vi "UHR-Fleezers Control (host) - 11.8.vi"() -> ()   [LabVIEW 2014] (continued)
        n1091 = Or(x="+ phase (APD Acq)", y="- phase (APD Acq)") -> (x .or. y?=w1470:bool)
        n1092 = xnode "Read/Write Control"("FPGA VI Reference In"=w1477, "error in"=w1476, "Phase Count Adjustment (APD Acq)"=w1474) -> ("FPGA VI Reference Out"=w1472:T19, "error out"=w1473:errorcluster)
        n1093 = xnode "Read/Write Control"("FPGA VI Reference In"=w1472, "error in"=w1473, "+ phase (APD Acq)"=w1470) -> ("error out"=w1471:errorcluster)  [unwired: 1 out]
      }
      event "Phase adj. (GI)", "+ phase (GI)", "- phase (GI)": Value Change {
        n1094 = event-data() -> ()  [unwired: 7 out]
        n1095 = Negate(x="Phase adj. (GI)") -> (-x=w1486:i16)
        n1096 = Select(t=w1486, s="+ phase (GI)", f="Phase adj. (GI)") -> (s? t:f=w1485:i16)
        n1097 = Or(x="+ phase (GI)", y="- phase (GI)") -> (x .or. y?=w1481:bool)
        n1098 = xnode "Read/Write Control"("FPGA VI Reference In"=w1488, "error in"=w1487, "Phase count adjustment (GI)"=w1485) -> ("FPGA VI Reference Out"=w1483:T19, "error out"=w1484:errorcluster)
        n1099 = xnode "Read/Write Control"("FPGA VI Reference In"=w1483, "error in"=w1484, "+ phase (GI)"=w1481) -> ("error out"=w1482:errorcluster)  [unwired: 1 out]
      }
      event "Phase adj. (GI) 2", "+ phase (GI) 2", "- phase (GI) 2": Value Change {
        n1100 = event-data() -> ()  [unwired: 7 out]
        n1101 = Negate(x="Phase adj. (GI) 2") -> (-x=w1497:i16)
        n1102 = Select(t=w1497, s="+ phase (GI) 2", f="Phase adj. (GI) 2") -> (s? t:f=w1496:i16)
        n1103 = Or(x="+ phase (GI) 2", y="- phase (GI) 2") -> (x .or. y?=w1492:bool)
        n1104 = xnode "Read/Write Control"("FPGA VI Reference In"=w1499, "error in"=w1498, "Phase count adjustment (GI) 2"=w1496) -> ("FPGA VI Reference Out"=w1494:T19, "error out"=w1495:errorcluster)
        n1105 = xnode "Read/Write Control"("FPGA VI Reference In"=w1494, "error in"=w1495, "+ phase (GI) 2"=w1492) -> ("error out"=w1493:errorcluster)  [unwired: 1 out]
      }
      event "Phase adj. (Green FB)", "- phase (Green FB)", "+ phase (Green FB)": Value Change {
        n1106 = event-data() -> ()  [unwired: 7 out]
        n1107 = Negate(x="Phase adj. (Green FB)") -> (-x=w1508:i16)
        n1108 = Select(t=w1508, s="+ phase (Green FB)", f="Phase adj. (Green FB)") -> (s? t:f=w1507:i16)
        n1109 = Or(x="+ phase (Green FB)", y="- phase (Green FB)") -> (x .or. y?=w1503:bool)
        n1110 = xnode "Read/Write Control"("FPGA VI Reference In"=w1510, "error in"=w1509, "Phase count adjustment (Green FB)"=w1507) -> ("FPGA VI Reference Out"=w1505:T19, "error out"=w1506:errorcluster)
        n1111 = xnode "Read/Write Control"("FPGA VI Reference In"=w1505, "error in"=w1506, "+ phase (Green FB)"=w1503) -> ("error out"=w1504:errorcluster)  [unwired: 1 out]
      }
      event "Invert APD Gate", "APD Gate ON Count", "APD Gate OFF Count", "APD Gate", "APD Integration Time (s)", "APD 1 AO Mult.", "APD 2 AO Mult.", "On one out of X cycles": Value Change {
        n1112 = event-data() -> ()  [unwired: 7 out]
        n1113 = Add(x="GI Frequency, ON count", y="GI Frequency, OFF count") -> (x+y=w1514:u32)
        n1114 = Add(x="APD Gate ON Count", y="APD Gate OFF Count") -> (x+y=w1527:u32)
        n1115 = Multiply(x="On one out of X cycles", y=w1514) -> (x*y=w1511:u32)
        "Green FB Count" <- w1511
        n1116 = Subtract(x=w1511, y="GI Frequency, ON count") -> (x-y=w1512:u32)
        n1117 = Multiply(x=w1527, y="On one out of X cycles") -> (x*y=w1526:u32)
        n1118 = Subtract(x=w1526, y="APD Gate ON Count") -> (x-y=w1525:u32)
        n1119 = local read "DMA Update Period (s)"() -> (w1528:dbl)
        n1120 = Multiply(x="APD Integration Time (s)", y=40000000.0) -> (x*y=w1533:dbl)
        n1121 = Reciprocal(x="APD Integration Time (s)") -> (1/x=→"APD Acq Rate (Hz)":dbl)
        n1122 = To Unsigned Long Integer(number=w1533) -> (unsigned 32bit integer=w1517:u32)
        "APD Int. Count" <- w1517
        n1123 = xnode "Read/Write Control"("FPGA VI Reference In"=w1537, "error in"=w1536, "Invert APD Gate"="Invert APD Gate", "APD Gate ON Count"="APD Gate ON Count", "APD Gate OFF Count"=w1525, "APD Acq Rate Count"=w1517, "APD Gate Operating Mode"="APD Gate", "APD 1 AO scale factor"="APD 1 AO Mult.", "APD 2 AO scale factor"="APD 2 AO Mult.", "Green interlace ON count"="GI Frequency, ON count", "Green interlace OFF count"=w1512, "Green interlace ON count 2"="GI Frequency, ON count", "Green interlace OFF count 2"=w1512, "Green FB Count"=w1511) -> ("error out"=w1535:errorcluster)  [unwired: 1 out]
        n1124 = Divide(x=w1528, y="APD Integration Time (s)") -> (x/y=w1531:dbl)
        n1125 = Multiply(x=2.0, y=w1531) -> (x*y=w1530:dbl)
        n1126 = local write "APD Samples/FIFO Acq."(w1531) -> ()
        n1127 = local write "APD Elements/DMA read"(w1530) -> ()
      }
      event "Number of F/B Scans (AOD)", "Scan Speed (nm/s)", "Scan BD", "Initial D (MHz)", "Step Size (nm)", "Scan Range (nm)", "Wiggle amp 1 (units?)": Value Change {
        w1599 = 123.0  # AOM cal (nm/MHz)
        n1128 = event-data() -> ()  [unwired: 7 out]
        n1129 = local read "BD 1 Frequency 1 (MHz)"() -> (w1582:dbl)
        n1130 = local read "AOM X Cal (nm/MHz)"() -> (w1574:dbl)
        n1131 = local read "BD 2 Frequency 1 (MHz)"() -> (w1588:dbl)
        n1132 = local read "X RF Frequency Limits (MHz)"() -> (w1586:T16)
        n1133 = local read "Y RF Frequency Limits (MHz)"() -> (w1583:T16)
        n1134 = Negate(x="Scan Range (nm)") -> (-x=w1552:dbl)
        n1135 = Divide(x=w1552, y=w1574) -> (x/y=w1556:dbl)
        n1136 = Select(t=w1586, s="Scan BD", f=w1583) -> (s? t:f=w1585:T16)
        n1137 = Select(t=w1582, s="Scan BD", f=w1588) -> (s? t:f=w1587:dbl)
        n1138 = Unbundle By Name(w1585) -> ("Maximum"=w1594:dbl, "Minimum"=w1593:dbl)
        n1139 = Add(x=w1556, y=w1587) -> (x+y=w1591:dbl)
        n1140 = Divide(x=w1552, y="Step Size (nm)") -> (x/y=w1571:dbl)
        n1141 = Divide(x="Step Size (nm)", y=w1574) -> (x/y=w1580:dbl)
        n1142 = Absolute Value(x=w1571) -> (abs(x)=w1555:dbl)
        n1143 = Sign(1:w1552) -> (0:w1553:dbl)
        n1144 = In Range and Coerce(upper limit=w1594, x=w1591, lower limit=w1593) -> (coerced(x)=w1590:dbl, In Range?=w1592:bool)
        n1145 = To Unsigned Quad Integer(1:w1555) -> (0:w1570:u64)
        "Scan steps (AOD)" <- w1570
        n1146 = call "IR AOM freq to word.vi"("Frequency In (MHz)"=w1580) -> ("Frequency Word Out (double)"=w1577:dbl)
        n1147 = Multiply(x=w1553, y=w1577) -> (x*y=w1554:dbl)
        n1148 = Subtract(x=w1591, y=w1590) -> (x-y=w1589:dbl)
        n1149 = To Quad Integer(1:w1554) -> (0:w1576:i64)
        "Incr. int (AOD)" <- w1576
        n1150 = Subtract(x=w1556, y=w1589) -> (x-y=w1575:dbl)
        "Scan Range (MHz)" <- w1575
        n1151 = Select(t=w1556, s=w1592, f=w1575) -> (s? t:f=w1595:dbl)
        n1152 = Multiply(x=w1575, y=w1574) -> (x*y=w1573:dbl)
        n1153 = Decrement(x=w1570) -> (x-1=w1623:u64)
        n1154 = Negate(x=w1573) -> (-x=w1569:dbl)
        n1155 = local write "Scan Range (nm)"(w1569) -> ()
        n1156 = Divide(x=w1595, y=w1623) -> (x/y=w1579:dbl)
        "Scan Increment (MHz)" <- w1579
        n1157 = call "IR AOM freq to word.vi"("Frequency In (MHz)"=w1579) -> ("Frequency Word Out (double)"=w1578:dbl)
        n1158 = Divide(x="Step Size (nm)", y="Scan Speed (nm/s)") -> (x/y=w1566:dbl)
        n1159 = To Quad Integer(1:w1578) -> ()  [unwired: 1 out]
        n1160 = local read "Number Interlace Sets"() -> (w1550:u8)
        n1161 = local read "AI Count (ticks)"() -> (w1551:u32)
        n1162 = local read "Total Counts (ticks)"() -> (w1549:u32)
        n1163 = local read "# Samples/trap"() -> (w1581:u32)
        n1164 = Multiply(x=w1551, y=w1550) -> (x*y=w1548:u32)
        n1165 = Divide(x=w1549, y=w1548) -> (x/y=w1547:dbl)
        n1166 = Select(t=w1582, s="Scan BD", f=w1588) -> (s? t:f=w1620:dbl)
        "Initial freq. (MHz)" <- w1620
        n1167 = Add(x=w1595, y=w1620) -> (x+y=→"Final freq. (MHz)":dbl)
        n1168 = Divide(x=w1549, y=40000000.0) -> (x/y=w1565:dbl)
        n1169 = Divide(x=w1566, y=w1565) -> (x/y=w1564:dbl)
        n1170 = To Unsigned Quad Integer(1:w1564) -> (0:w1539:u64)
        n1171 = Quotient & Remainder(x=w1539, y=u64 2) -> (x-y*floor(x/y)=w1543:u64)  [unwired: 1 out]
        n1172 = Equal?(x=w1543, y=u64 0) -> (x = y?=w1541:bool)
        n1173 = Decrement(x=w1539) -> (x-1=w1540:u64)
        n1174 = Select(t=w1539, s=w1541, f=w1540) -> (s? t:f=w1538:u64)
        "Cycles/step (AOD)" <- w1538
        n1175 = xnode "Read/Write Control"("FPGA VI Reference In"=w1631, "error in"=w1630, "Scan steps"=w1570, "Number of scans"="Number of F/B Scans (AOD)", "Cycles per step"=w1538, "Scan freq.  increment"=w1576, "Scan BD"="Scan BD") -> ("error out"=w1629:errorcluster)  [unwired: 1 out]
        n1176 = Multiply(x=w1570, y=w1538) -> (x*y=w1624:u64)
        n1177 = Multiply(x=w1624, y=u64 2) -> (x*y=w1546:u64)
        n1178 = Multiply(x=w1547, y=w1546) -> (x*y=w1545:dbl)
        "Data points/scan (f/b)" <- w1545
        n1179 = Multiply(x=w1545, y="Number of F/B Scans (AOD)") -> (x*y=w1627:dbl)
        "Data points/scans" <- w1627
        n1180 = Divide(x=w1627, y=w1581) -> (x/y=→"N sets should be saved":dbl)
        n1181 = Multiply(x=w1624, y=w1565) -> (x*y=w1563:dbl)
        "Time/Scan (s) (AOD)" <- w1563
        n1182 = Select(t=w1595, s="Scan BD", f=0.0) -> (s? t:f=w1621:dbl)
        n1183 = Select(t=0.0, s="Scan BD", f=w1595) -> (s? t:f=w1617:dbl)
        n1184 = local read "BD 2 Frequency 2 (MHz)"() -> (w1613:dbl)
        n1185 = local read "BD 1 Frequency 2 (MHz)"() -> (w1616:dbl)
        n1186 = Add(x=w1617, y=w1588) -> (x+y=w1614:dbl)
        n1187 = Add(x=w1582, y=w1621) -> (x+y=w1615:dbl)
        n1188 = Multiply(x=w1563, y=2.0) -> (x*y=w1562:dbl)
        n1189 = Multiply(x=w1562, y="Number of F/B Scans (AOD)") -> (x*y=w1559:dbl)
        n1190 = Divide(x=w1559, y=60.0) -> (x/y=→"Time to Finish All (min)":dbl)
        n1191 = Add(x="Trap 2 Bead Size (nm)", y="Trap 1 Bead Size (nm)") -> (x+y=w1603:dbl)
        n1192 = Divide(x=w1603, y=2.0) -> (x/y=w1597:dbl)
        n1193 = Subtract(x=w1614, y=w1613) -> (x-y=w1611:dbl)
        n1194 = Subtract(x=w1615, y=w1616) -> (x-y=w1612:dbl)
        n1195 = local read "Initial D (MHz)"() -> (w1600:dbl)
        n1196 = Square(x=w1611) -> (x^2=w1610:dbl)
        n1197 = Square(x=w1612) -> (x^2=w1609:dbl)
        n1198 = Add(x=w1609, y=w1610) -> (x+y=w1608:dbl)
        n1199 = Square Root(x=w1608) -> (sqrt(x)=w1607:dbl)
        "Final D (MHz)" <- w1607
        n1200 = Multiply(x=w1599, y=w1607) -> (x*y=w1606:dbl)
        n1201 = Multiply(x=w1600, y=w1599) -> (x*y=w1598:dbl)
        n1202 = Subtract(x=w1598, y=w1597) -> (x-y=→"Initial sep (nm)":dbl)
        n1203 = Subtract(x=w1606, y=w1597) -> (x-y=→"Final sep (nm)":dbl)
      }
      event "Freq or Amp switch first", "Swap F1 and F2", "Freq switch delay", "Amp switch delay": Value Change {
        n1204 = event-data() -> ()  [unwired: 7 out]
        n1205 = local read "Freq or Amp switch first"() -> (w1632:bool)
        n1206 = local read "Amp switch delay"() -> (w1633:u16)
        n1207 = local read "Freq switch delay"() -> (w1635:u16)
        n1208 = local read "Swap F1 and F2"() -> (w1634:bool)
        n1209 = xnode "Read/Write Control"("FPGA VI Reference In"=w1638, "error in"=w1637, "Freq switch delay"=w1635, "Swap F1 and F2"=w1634, "Amp switch delay"=w1633, "Freq or Amp switch first"=w1632) -> ("error out"=w1636:errorcluster)  [unwired: 1 out]
      }
      event "Scan steps (MCL)", "Number of scans (MCL)", "Scan Range (V)\n(of steps)", "2D or 1D Scan", "N APD Samp/step", "Fast Scan Dir", "Continuous MCL Scanning", "Scan lines (y)": Value Change {
        w1640 = 32767.0 ("y")
        n1210 = event-data() -> ()  [unwired: 7 out]
        n1211 = Select(t="Scan lines (y)", s="2D or 1D Scan", f="Number of scans (MCL)") -> (s? t:f=w1645:u64)
        n1212 = Decrement(x="Scan steps (MCL)") -> (x-1=w1661:u64)
        n1213 = Divide(x="Scan Range (V)\n(of steps)", y=w1661) -> (x/y=w1660:dbl)
        "Desired Scan Incr (V)" <- w1660
        n1214 = local read "APD Integration Time (s)"() -> (w1653:dbl)
        n1215 = Multiply(x=w1660, y=w1640) -> (x*y=w1669:dbl)
        n1216 = Divide(x=w1669, y=10.0) -> (x/y=w1659:dbl)
        "Desired incr (int)" <- w1659
        n1217 = local read "Update Count (MCL)"() -> (w1665:u32)
        n1218 = Round Toward -Infinity(1:w1659) -> (0:w1668:dbl)
        n1219 = To Word Integer(number=w1668) -> (16bit integer=w1643:i16)
        "Actual Incr. int (MCL)" <- w1643
        n1220 = Multiply(x=w1653, y=40000000.0) -> (x*y=w1666:dbl)
        n1221 = Divide(x=w1666, y=w1665) -> (x/y=w1664:dbl)
        n1222 = Multiply(x=i16 10, y=w1643) -> (x*y=w1641:i16)
        n1223 = Multiply(x="N APD Samp/step", y=w1664) -> (x*y=w1663:dbl)
        "Cycles/step (MCL)" <- w1663
        n1224 = Divide(x=w1641, y=w1640) -> (x/y=→"Actual MCL Inc (V)":dbl)
        n1225 = Multiply(x="N APD Samp/step", y="Scan steps (MCL)") -> (x*y=w1655:dbl)
        n1226 = local read "APD Samples/FIFO Acq."() -> (w1652:dbl)
        n1227 = Multiply(x=w1655, y=u64 2) -> (x*y=w1654:dbl)
        "Data points/scan (f+b)" <- w1654
        n1228 = Multiply(x=w1654, y=w1645) -> (x*y=w1672:dbl)
        "Data points/scans (MCL)" <- w1672
        n1229 = Multiply(x=w1653, y=w1654) -> (x*y=w1646:dbl)
        "Time/f+b scan (s) (MCL)" <- w1646
        n1230 = Divide(x=w1672, y=w1652) -> (x/y=→"N sets should be saved (MCL)":dbl)
        n1231 = Multiply(x=w1646, y=w1645) -> (x*y=→"Total Time (s)":dbl)
        n1232 = Not(x="Fast Scan Dir") -> (.not. x?=w1650:bool)
        n1233 = xnode "Read/Write Control"("FPGA VI Reference In"=w1676, "error in"=w1675, "Scan steps (MCL)"="Scan steps (MCL)", "Number of scans (MCL)"=w1645, "Cycles per step (MCL)"=w1663, "Scan freq.  increment (MCL)"=w1643, "1D or 2D Scan?"="2D or 1D Scan", "MCL Scan Axis"=w1650, "Cont. Scan (MCL)"="Continuous MCL Scanning") -> ("error out"=w1674:errorcluster)  [unwired: 1 out]
      }
      event "Read Cal": Value Change {
        w1678 = 1000.0 ("y")
        n1234 = event-data() -> ()  [unwired: 7 out]
        n1235 = local read "Save file name"() -> (w1703:path)
        n1236 = local write "Read Cal"(FALSE ("Read Cal")) -> ()
        n1237 = Strip Path(path=w1703) -> (stripped path=w1702:path)  [unwired: 1 out]
        n1238 = Path To String(path=w1702) -> (string=w1701:string)
        n1239 = Concatenate Strings(w1701, "\\current.cal" ("string")) -> (w1699:string)
        n1240 = String To Path(string=w1699) -> (path=w1698:path)
        n1241 = Open/Create/Replace File(file path (use dialog)=w1698, operation (0:open)=T25."open", access (0:read/write)=enum16{"read/write", "read-only", "write-only"}."read-only") -> (refnum out=w1706:refnum<file>, error out=w1692:errorcluster)  [unwired: 1 in, 3 out]
        n1242 = Deny Access(4:w1692, 7:w1706) -> (0:w1691:errorcluster, 3:w1697:refnum<file>)  [unwired: 1 out]
        n1243 = Read from Binary File(5:0.0, 8:w1691, 9:T24."big-endian, network order" ("byte order (0:big-endian, network order)"), 10:-1 ("count (1)"), 11:w1697) -> (0:w1690:errorcluster, 2:w1688:dbl[], 3:w1693:refnum<file>)  [unwired: 2 out]
        n1244 = Array To Cluster(array=w1688) -> (cluster=w1687:T27)
        n1245 = Unbundle(w1687) -> ("[0]"=w1686:dbl, "[1]"=w1685:dbl, "[2]"=w1684:dbl, "[3]"=w1683:dbl, "[4]"=w1682:dbl, "[5]"=w1681:dbl)
        n1246 = Close File(refnum=w1693, error in=w1690) -> (error out=→"Read cal error":errorcluster)  [unwired: 1 out]
        n1247 = Multiply(x=w1681, y=w1678) -> (x*y=w1679:dbl)
        n1248 = local write "T2 k_x (pN/nm)"(w1683) -> ()
        n1249 = local write "T1 k_x (pN/nm)"(w1684) -> ()
        n1250 = local write "T1 a_x (nm/V)"(w1686) -> ()
        n1251 = local write "T2 a_x (nm/V)"(w1685) -> ()
        n1252 = Multiply(x=w1682, y=w1678) -> (x*y=w1680:dbl)
        n1253 = local write "T1 offset_x (mV)"(w1680) -> ()
        n1254 = local write "T2 offset_x (mV)"(w1679) -> ()
      }
      event "Read FX file": Value Change {
        n1255 = event-data() -> ()  [unwired: 7 out]
        n1256 = local write "Read FX file"(FALSE ("Read residual")) -> ()
        n1257 = local read "Save file name"() -> (w1731:path)
        n1258 = Strip Path(path=w1731) -> (stripped path=w1730:path)  [unwired: 1 out]
        n1259 = Path To String(path=w1730) -> (string=w1729:string)
        n1260 = Concatenate Strings(w1729, "\\current.cal" ("string")) -> (w1727:string)
        n1261 = String To Path(string=w1727) -> (path=w1726:path)
        n1262 = Open/Create/Replace File(file path (use dialog)=w1726, operation (0:open)=T25."open", access (0:read/write)=enum16{"read/write", "read-only", "write-only"}."read-only") -> (refnum out=w1723:refnum<file>, error out=w1720:errorcluster)  [unwired: 3 in, 1 out]
        n1263 = Deny Access(4:w1720, 7:w1723) -> (0:w1719:errorcluster, 3:w1722:refnum<file>)  [unwired: 1 in]
        n1264 = Read from Binary File(5:0.0, 8:w1719, 9:T24."big-endian, network order" ("byte order (0:big-endian, network order)"), 10:-1 ("count"), 11:w1722) -> (0:w1715:errorcluster, 2:w1709:dbl[], 3:w1716:refnum<file>)  [unwired: 1 in, 1 out]
        n1265 = Index Array(array=w1709, index=6) -> (element=→"Bad fit error":dbl)
        n1266 = Index Array(array=w1709, index=7) -> (element=→"Fit offset":dbl)
        n1267 = Index Array(array=w1709, index=8) -> (element=→"Hyst. error":dbl)
        n1268 = Close File(refnum=w1716, error in=w1715) -> ()  [unwired: 2 out]
      }
      event "Abort MCL Scan": Value Change {
        n1269 = event-data() -> ()  [unwired: 7 out]
        n1270 = local write "MCL Scanning"(FALSE ("MCL Scanning")) -> ()
        n1271 = xnode "Read/Write Control"("FPGA VI Reference In"=w1736, "error in"=w1735, "Abort scan (MCL)"="Abort MCL Scan") -> ("error out"=w1734:errorcluster)  [unwired: 1 out]
      }
      event "Update Count (MCL)": Value Change {
        n1272 = event-data() -> ()  [unwired: 7 out]
        n1273 = xnode "Read/Write Control"("FPGA VI Reference In"=w1740, "error in"=w1739, "MCL count"="Update Count (MCL)") -> ("error out"=w1738:errorcluster)  [unwired: 1 out]
      }
      event "Phase adjust (MCL)", "+ phase (MCL)", "- phase (MCL)": Value Change {
        n1274 = event-data() -> ()  [unwired: 7 out]
        n1275 = Negate(x="Phase adjust (MCL)") -> (-x=w1749:i16)
        n1276 = Select(t=w1749, s="- phase (MCL)", f="Phase adjust (MCL)") -> (s? t:f=w1747:i16)
        n1277 = Or(x="- phase (MCL)", y="+ phase (MCL)") -> (x .or. y?=w1742:bool)
        n1278 = xnode "Read/Write Control"("FPGA VI Reference In"=w1751, "error in"=w1750, "Phase count adjustment (MCL)"=w1747) -> ("FPGA VI Reference Out"=w1743:T19, "error out"=w1744:errorcluster)
        n1279 = xnode "Read/Write Control"("FPGA VI Reference In"=w1743, "error in"=w1744, "+ phase (MCL)"=w1742) -> ("error out"=w1741:errorcluster)  [unwired: 1 out]
      }
      event "Abort AOD Scan": Value Change {
        n1280 = event-data() -> ()  [unwired: 7 out]
        n1281 = xnode "Read/Write Control"("FPGA VI Reference In"=w1755, "error in"=w1754, "Abort scan"="Abort AOD Scan") -> ("error out"=w1753:errorcluster)  [unwired: 1 out]
      }
      event "Continuous AOD Scanning": Value Change {
        n1282 = event-data() -> ()  [unwired: 7 out]
        n1283 = xnode "Read/Write Control"("FPGA VI Reference In"=w1759, "error in"=w1758, "Cont. Scan"="Continuous AOD Scanning") -> ("error out"=w1757:errorcluster)  [unwired: 1 out]
      }
      event "Index": Value Change {
        n1284 = event-data() -> ()  [unwired: 7 out]
        n1285 = call "Create new save file.vi"("Insert"="", "Ext"=".dat" ("string"), "Index In"="Index") -> ("Path Out"=→"Save file name":path, "Index Out"=w1760:dbl)
        "Save index" <- w1760
        n1286 = local write "Index"(w1760) -> ()
      }
      event "AO1", "AO2": Value Change {
        w1775 = 10.0 ("y")
        w1774 = 32767.0 ("y")
        n1287 = event-data() -> ()  [unwired: 7 out]
        n1288 = local read "AO2"() -> (w1773:dbl)
        n1289 = local read "AO1"() -> (w1770:dbl)
        n1290 = Multiply(x=w1770, y=w1774) -> (x*y=w1769:dbl)
        n1291 = Multiply(x=w1773, y=w1774) -> (x*y=w1772:dbl)
        n1292 = Divide(x=w1769, y=w1775) -> (x/y=w1768:dbl)
        n1293 = Divide(x=w1772, y=w1775) -> (x/y=w1771:dbl)
        n1294 = To Word Integer(number=w1768) -> (16bit integer=w1776:i16)
        n1295 = To Word Integer(number=w1771) -> (16bit integer=w1777:i16)
        n1296 = xnode "Read/Write Control"("FPGA VI Reference In"=w1767, "error in"=w1766, "AO1"=w1776, "AO2"=w1777) -> ("error out"=w1765:errorcluster)  [unwired: 1 out]
      }
      event "Inject Pump 1": Value Change {
        n1297 = event-data() -> ()  [unwired: 7 out]
        n1298 = local read "Use Harvard pumps\nfor beads (else Chemyx)"() -> (w1779:bool)
        n1299 = case shown="True" w1779 {
          tunnel: "Inject Pump 1" -> [w1783 w1821]
          tunnel: w1778 -> [_ w1822]
          frame False {
            n1300 = local read "Pump write delay (ms)"() -> (w1782:dbl)
            n1301 = local read "Chemyx Syringe Pump Serial Port"() -> (w1781:refnum<visa-resource-name>)
            n1302 = case shown="True" w1783 {
              tunnel: w1782 -> [w1789 w1803]
              tunnel: w1781 -> [w1786 w1802]
              frame False {
                n1303 = flat-sequence {
                  tunnel: w1786 -> [w1790]
                  tunnel: [w1790] -> w1787
                  tunnel: w1789 -> [_]
                  tunnel: [w1793] -> w1788
                  tunnel: w1787 -> [w1793]
                  tunnel: w1788 -> [w1794]
                  tunnel: [w1794] -> w1784
                  tunnel: [w1796] -> w1785
                  tunnel: w1784 -> [w1796]
                  tunnel: w1785 -> [w1798]
                  frame #0 {
                    n1304 = call "Write to pump.vi"("string"="enter pump1", "VISA resource name"=w1790) -> ()  [unwired: 1 out]
                  }
                  frame #1 {
                    n1305 = Wait (ms)(milliseconds to wait="Pump pause delay (ms)") -> ()  [unwired: 1 out]
                  }
                  frame #2 {
                    n1306 = call "Write to pump.vi"("string"="stop", "VISA resource name"=w1794) -> ()  [unwired: 1 out]
                  }
                  frame #3 {
                    n1307 = Wait (ms)(milliseconds to wait=u32 500) -> ()  [unwired: 1 out]
                  }
                  frame #4 {
                    n1308 = call "Write to pump.vi"("string"="stop", "VISA resource name"=w1798) -> ()  [unwired: 1 out]
                  }
                }
              }
              frame True {
                n1309 = flat-sequence {
                  tunnel: w1802 -> [w1812]
                  tunnel: w1803 -> [w1807]
                  tunnel: w1803 -> [w1814]
                  tunnel: w1802 -> [w1815]
                  tunnel: [w1815] -> w1800
                  tunnel: [w1817] -> w1801
                  tunnel: w1800 -> [w1817]
                  tunnel: w1801 -> [w1819]
                  frame #0 {
                    n1310 = local read "All Pump Parameters"() -> (w1806:T5)
                    n1311 = Unbundle By Name(w1806) -> ("Pump 1"=w1813:T28)
                    n1312 = call "Set pump parameters.vi"("Pump write delay (ms)"=w1807, "Volume (uL)"="Ch 1 Inject Volume (uL)", "Rate (uL/h)"="Ch 1 Inject Rate (ul/h)", "Units"=4.0, "Pump #"=1.0, "Pump Parameters In"=w1813, "VISA resource name"=w1812) -> ("Pump Parameters Out"=w1805:T28)  [unwired: 3 in]
                    n1313 = Bundle By Name(cluster=w1806, "Pump 1"=w1805) -> (w1804:T5)
                    n1314 = local write "All Pump Parameters"(w1804) -> ()
                  }
                  frame #1 {
                    n1315 = Wait (ms)(milliseconds to wait=w1814) -> ()  [unwired: 1 out]
                  }
                  frame #2 {
                    n1316 = call "Write to pump.vi"("string"="start", "VISA resource name"=w1815) -> ()  [unwired: 1 out]
                  }
                  frame #3 {
                    n1317 = Wait (ms)(milliseconds to wait=u32 500) -> ()  [unwired: 1 out]
                  }
                  frame #4 {
                    n1318 = call "Write to pump.vi"("string"="start", "VISA resource name"=w1819) -> ()  [unwired: 1 out]
                  }
                }
              }
            }
          }
          frame True {
            n1319 = case shown="True" w1821 {
              tunnel: w1822 -> [w1823 w1833]
              frame False {
                n1320 = flat-sequence {
                  tunnel: w1823 -> [w1825]
                  frame #0 {
                    n1321 = local write "Flushing P1"(FALSE ("Flushing P1")) -> ()
                    n1322 = Concatenate Strings("stop" ("string"), "\r") -> (w1827:string)
                    n1323 = VISA Write(VISA resource name=w1825, write buffer=w1827) -> ()  [unwired: 1 in, 3 out]
                  }
                  frame #1 {
                    n1324 = property on="Clear Volume P1" class="Bool (strict)"("Val(Sgnl)"=TRUE ("Value (Signaling)")) -> ()  [unwired: 2 in, 2 out]
                  }
                }
              }
              frame True {
                n1325 = local read "Normal Flow Rate (ul/h) P1"() -> (w1831:dbl)
                n1326 = Number To Decimal String(number=w1831) -> (decimal integer string=w1837:string)  [unwired: 1 in]
                n1327 = Concatenate Strings("irate  " ("string"), w1837, " u/h" ("string"), "\r") -> (w1835:string)
                n1328 = VISA Write(VISA resource name=w1833, write buffer=w1835) -> (VISA resource name out=w1832:refnum<visa-resource-name>)  [unwired: 1 in, 2 out]
                n1329 = Concatenate Strings("irun" ("string"), "\r") -> (w1839:string)
                n1330 = VISA Write(VISA resource name=w1832, write buffer=w1839) -> ()  [unwired: 1 in, 3 out]
              }
            }
          }
        }
      }
      event "Inject Pump 3": Value Change {
        n1331 = event-data() -> ()  [unwired: 7 out]
        n1332 = local read "Use Harvard pumps\nfor beads (else Chemyx)"() -> (w1842:bool)
        n1333 = case shown="True" w1842 {
          tunnel: "Inject Pump 3" -> [w1846 w1885]
          tunnel: w1841 -> [_ w1884]
          frame False {
            n1334 = local read "Pump write delay (ms)"() -> (w1845:dbl)
            n1335 = case shown="True" w1846 {
              tunnel: w1845 -> [w1852 w1866]
              tunnel: "Chemyx Syringe Pump Serial Port" -> [w1849 w1865]
              frame False {
                n1336 = flat-sequence {
                  tunnel: w1849 -> [w1853]
                  tunnel: [w1853] -> w1850
                  tunnel: w1852 -> [_]
                  tunnel: [w1856] -> w1851
                  tunnel: w1850 -> [w1856]
                  tunnel: w1851 -> [w1857]
                  tunnel: [w1857] -> w1847
                  tunnel: [w1859] -> w1848
                  tunnel: w1847 -> [w1859]
                  tunnel: w1848 -> [w1861]
                  frame #0 {
                    n1337 = call "Write to pump.vi"("string"="enter pump3", "VISA resource name"=w1853) -> ()  [unwired: 1 out]
                  }
                  frame #1 {
                    n1338 = local read "Pump pause delay (ms)"() -> (w1855:u32)
                    n1339 = Wait (ms)(milliseconds to wait=w1855) -> ()  [unwired: 1 out]
                  }
                  frame #2 {
                    n1340 = call "Write to pump.vi"("string"="stop", "VISA resource name"=w1857) -> ()  [unwired: 1 out]
                  }
                  frame #3 {
                    n1341 = Wait (ms)(milliseconds to wait=u32 0) -> ()  [unwired: 1 out]
                  }
                  frame #4 {
                    n1342 = call "Write to pump.vi"("string"="stop", "VISA resource name"=w1861) -> ()  [unwired: 1 out]
                  }
                }
              }
              frame True {
                n1343 = flat-sequence {
                  tunnel: w1865 -> [w1875]
                  tunnel: w1866 -> [w1870]
                  tunnel: w1866 -> [w1877]
                  tunnel: w1865 -> [w1878]
                  tunnel: [w1878] -> w1864
                  tunnel: [w1881] -> w1863
                  tunnel: w1864 -> [w1881]
                  tunnel: w1863 -> [w1882]
                  frame #0 {
                    n1344 = local read "All Pump Parameters"() -> (w1869:T5)
                    n1345 = Unbundle By Name(w1869) -> ("Pump 3"=w1876:T28)
                    n1346 = call "Set pump parameters.vi"("Pump write delay (ms)"=w1870, "Volume (uL)"="Ch 3 Inject Volume (uL)", "Rate (uL/h)"="Ch 3 Inject Rate (ul/h)", "Units"=4.0, "Pump #"=3.0, "Pump Parameters In"=w1876, "VISA resource name"=w1875) -> ("Pump Parameters Out"=w1868:T28)  [unwired: 3 in]
                    n1347 = Bundle By Name(cluster=w1869, "Pump 3"=w1868) -> (w1867:T5)
                    n1348 = local write "All Pump Parameters"(w1867) -> ()
                  }
                  frame #1 {
                    n1349 = Wait (ms)(milliseconds to wait=w1877) -> ()  [unwired: 1 out]
                  }
                  frame #2 {
                    n1350 = call "Write to pump.vi"("string"="start", "VISA resource name"=w1878) -> ()  [unwired: 1 out]
                  }
                  frame #3 {
                    n1351 = Wait (ms)(milliseconds to wait=u32 500) -> ()  [unwired: 1 out]
                  }
                  frame #4 {
                    n1352 = call "Write to pump.vi"("string"="start", "VISA resource name"=w1882) -> ()  [unwired: 1 out]
                  }
                }
              }
            }
          }
          frame True {
            n1353 = case shown="True" w1885 {
              tunnel: w1884 -> [w1886 w1893]
              frame False {
                n1354 = flat-sequence {
                  tunnel: w1886 -> [w1888]
                  frame #0 {
                    n1355 = local write "Flushing P3"(FALSE ("Flushing P3")) -> ()
                    n1356 = Concatenate Strings("stop" ("string"), "\r") -> (w1890:string)
                    n1357 = VISA Write(VISA resource name=w1888, write buffer=w1890) -> ()  [unwired: 1 in, 3 out]
                  }
                  frame #1 {
                    n1358 = property on="Clear Volume P3" class="Bool (strict)"("Val(Sgnl)"=TRUE ("Value (Signaling)")) -> ()  [unwired: 2 in, 2 out]
                  }
                }
              }
              frame True {
                n1359 = local read "Normal Flow Rate (ul/h) P3"() -> (w1894:dbl)
                n1360 = Number To Decimal String(number=w1894) -> (decimal integer string=w1900:string)  [unwired: 1 in]
                n1361 = Concatenate Strings("irate  " ("string"), w1900, " u/h" ("string"), "\r") -> (w1898:string)
                n1362 = VISA Write(VISA resource name=w1893, write buffer=w1898) -> (VISA resource name out=w1896:refnum<visa-resource-name>)  [unwired: 1 in, 2 out]
                n1363 = Concatenate Strings("irun" ("string"), "\r") -> (w1902:string)
                n1364 = VISA Write(VISA resource name=w1896, write buffer=w1902) -> ()  [unwired: 1 in, 3 out]
              }
            }
          }
        }
      }
      event "Inject Pump 2": Value Change {
        n1365 = event-data() -> ()  [unwired: 7 out]
        n1366 = local read "Pump write delay (ms)"() -> (w1906:dbl)
        n1367 = local read "Chemyx Syringe Pump Serial Port"() -> (w1904:refnum<visa-resource-name>)
        n1368 = flat-sequence {
          tunnel: w1904 -> [w1919]
          tunnel: w1906 -> [w1915]
          tunnel: "Inject Pump 2" -> [_]
          tunnel: w1906 -> [w1921]
          tunnel: w1904 -> [w1922]
          frame #0 {
            n1369 = local read "All Pump Parameters"() -> (w1914:T5)
            n1370 = Multiply(x=60.0, y="Flush Center Ch Rate (ul/m)") -> (x*y=w1911:dbl)
            n1371 = Unbundle By Name(w1914) -> ("Pump 2"=w1920:T28)
            n1372 = call "Set pump parameters.vi"("Pump write delay (ms)"=w1915, "Volume (uL)"="Flush Center Ch Volume (uL)", "Rate (uL/h)"=w1911, "Units"=3.0, "Pump #"=2.0, "Pump Parameters In"=w1920, "VISA resource name"=w1919) -> ("Pump Parameters Out"=w1913:T28)  [unwired: 3 in]
            n1373 = Bundle By Name(cluster=w1914, "Pump 2"=w1913) -> (w1912:T5)
            n1374 = Add(x="Flush Center Ch Volume (uL)", y="Total Volume\nFlushed (uL)") -> (x+y=w1908:dbl)
            n1375 = local write "All Pump Parameters"(w1912) -> ()
            n1376 = local write "Total Volume\nFlushed (uL)"(w1908) -> ()
          }
          frame #1 {
            n1377 = Wait (ms)(milliseconds to wait=w1921) -> ()  [unwired: 1 out]
          }
          frame #2 {
            n1378 = call "Write to pump.vi"("string"="start", "VISA resource name"=w1922) -> ()  [unwired: 1 out]
          }
        }
      }
      event "Sample Channel\nFlow": Value Change {
        n1379 = event-data() -> ()  [unwired: 7 out]
        n1380 = case shown="True" "Sample Channel\nFlow" {
          tunnel: w1925 -> [w1926 w1932]
          frame False {
            n1381 = flat-sequence {
              tunnel: w1926 -> [w1928]
              frame #0 {
                n1382 = local write "Flushing samp"(FALSE ("Flushing samp")) -> ()
                n1383 = Concatenate Strings("stop" ("string"), "\r") -> (w1931:string)
                n1384 = VISA Write(VISA resource name=w1928, write buffer=w1931) -> ()  [unwired: 1 in, 3 out]
              }
            }
          }
          frame True {
            n1385 = local read "Normal Flow rate (mL/h)"() -> (w1942:dbl)
            n1386 = Number To Decimal String(number=w1942) -> (decimal integer string=w1941:string)  [unwired: 1 in]
            n1387 = Concatenate Strings("irate " ("string"), w1941, " u/h" ("string"), "\r") -> (w1937:string)
            n1388 = VISA Write(VISA resource name=w1932, write buffer=w1937) -> (VISA resource name out=w1936:refnum<visa-resource-name>)  [unwired: 1 in, 2 out]
            n1389 = Concatenate Strings("irun" ("string"), "\r") -> (w1933:string)
            n1390 = VISA Write(VISA resource name=w1936, write buffer=w1933) -> ()  [unwired: 1 in, 3 out]
          }
        }
      }
      event "Start Flow": Value Change {
        n1391 = event-data() -> ()  [unwired: 7 out]
        n1392 = local write "Sample Channel\nFlow"(TRUE ("Sample Channel\nFlow")) -> ()
        n1393 = local write "Start Flow"(FALSE ("Start Flow")) -> ()
        n1394 = Concatenate Strings("irun" ("string"), "\r") -> (w1947:string)
        n1395 = VISA Write(VISA resource name=w1943, write buffer=w1947) -> ()  [unwired: 1 in, 3 out]
      }
      event "Stop Flow": Value Change {
        w1949 = FALSE ("Stop Flow")
        n1396 = event-data() -> ()  [unwired: 7 out]
        n1397 = local write "Stop Flow"(w1949) -> ()
        n1398 = local write "Sample Channel\nFlow"(w1949) -> ()
        n1399 = Concatenate Strings("stop" ("string"), "\r") -> (w1952:string)
        n1400 = VISA Write(VISA resource name=w1950, write buffer=w1952) -> ()  [unwired: 1 in, 3 out]
      }
      event "Normal Flow rate (mL/h)": Value Change {
        n1401 = event-data() -> ()  [unwired: 7 out]
        n1402 = Number To Decimal String(number="Normal Flow rate (mL/h)") -> (decimal integer string=w1959:string)  [unwired: 1 in]
        n1403 = Concatenate Strings("irate  " ("string"), w1959, " u/h" ("string"), "\r") -> (w1958:string)
        n1404 = VISA Write(VISA resource name=w1955, write buffer=w1958) -> ()  [unwired: 1 in, 3 out]
      }
      event "Flush Sample": Value Change {
        n1405 = event-data() -> ()  [unwired: 7 out]
        n1406 = flat-sequence {
          tunnel: w1961 -> [w1989]
          frame #0 {
            # "set parameters (rate, volume) for flush, clear volume"
            n1407 = Number To Decimal String(number="Flush rate (mL/m)") -> (decimal integer string=w1985:string)  [unwired: 1 in]
            n1408 = local write "Sample Channel\nFlow"(TRUE ("Sample Channel\nFlow")) -> ()
            n1409 = Concatenate Strings("irate  " ("string"), w1985, " u/m" ("string"), "\r") -> (w1987:string)
            n1410 = VISA Write(VISA resource name=w1989, write buffer=w1987) -> (VISA resource name out=w1983:refnum<visa-resource-name>)  [unwired: 1 in, 2 out]
            n1411 = Number To Decimal String(number="Flush volume (mL)") -> (decimal integer string=w1974:string)  [unwired: 1 in]
            n1412 = Reciprocal(x="Flush rate (mL/m)") -> (1/x=w1968:dbl)
            n1413 = Concatenate Strings("tvolume  " ("string"), w1974, " u" ("string"), "\r") -> (w1972:string)
            n1414 = Multiply(x=w1968, y="Flush volume (mL)") -> (x*y=w1966:dbl)
            n1415 = VISA Write(VISA resource name=w1983, write buffer=w1972) -> (VISA resource name out=w1971:refnum<visa-resource-name>)  [unwired: 1 in, 2 out]
            n1416 = Multiply(x=w1966, y=60.0) -> (x*y=→"Samp Flush Time (s)":dbl)
            n1417 = Concatenate Strings("cvolume" ("string"), "\r") -> (w1970:string)
            n1418 = VISA Write(VISA resource name=w1971, write buffer=w1970) -> (VISA resource name out=w1981:refnum<visa-resource-name>)  [unwired: 1 in, 2 out]
            n1419 = Concatenate Strings("irun" ("string"), "\r") -> (w1979:string)
            n1420 = VISA Write(VISA resource name=w1981, write buffer=w1979) -> ()  [unwired: 1 in, 3 out]
          }
          frame #1 {
            "Flushing samp" <- TRUE ("Boolean")
          }
        }
      }
      event "Flush Pump 3": Value Change {
        n1421 = event-data() -> ()  [unwired: 7 out]
        n1422 = flat-sequence {
          tunnel: w1991 -> [w1994]
          frame #0 {
            # "set paramaters (rate, volume) for flush, clear volume"
            n1423 = Number To Decimal String(number="Flush rate (uL/m) P3") -> (decimal integer string=w2016:string)  [unwired: 1 in]
            n1424 = local write "Inject Pump 3"(TRUE ("Inject Pump 3")) -> ()
            n1425 = Concatenate Strings("irate  " ("string"), w2016, " u/m" ("string"), "\r") -> (w2018:string)
            n1426 = VISA Write(VISA resource name=w1994, write buffer=w2018) -> (VISA resource name out=w2014:refnum<visa-resource-name>)  [unwired: 1 in, 2 out]
            n1427 = Reciprocal(x="Flush rate (uL/m) P3") -> (1/x=w1998:dbl)
            n1428 = Number To Decimal String(number="Volume (uL) P3") -> (decimal integer string=w2005:string)  [unwired: 1 in]
            n1429 = Multiply(x="Volume (uL) P3", y=w1998) -> (x*y=w1997:dbl)
            n1430 = Concatenate Strings("tvolume  " ("string"), w2005, " u" ("string"), "\r") -> (w2003:string)
            n1431 = Multiply(x=w1997, y=60.0) -> (x*y=→"HP3 Flush Time (s)":dbl)
            n1432 = VISA Write(VISA resource name=w2014, write buffer=w2003) -> (VISA resource name out=w2002:refnum<visa-resource-name>)  [unwired: 1 in, 2 out]
            n1433 = Concatenate Strings("cvolume" ("string"), "\r") -> (w2001:string)
            n1434 = VISA Write(VISA resource name=w2002, write buffer=w2001) -> (VISA resource name out=w2012:refnum<visa-resource-name>)  [unwired: 1 in, 2 out]
            n1435 = Concatenate Strings("irun" ("string"), "\r") -> (w2010:string)
            n1436 = VISA Write(VISA resource name=w2012, write buffer=w2010) -> ()  [unwired: 1 in, 3 out]
          }
          frame #1 {
            "Flushing P3" <- TRUE ("Flushing P3")
          }
        }
      }
      event "Flush Pump 1": Value Change {
        n1437 = event-data() -> ()  [unwired: 7 out]
        n1438 = flat-sequence {
          tunnel: [w2032] -> w2022
          tunnel: w2021 -> [w2025]
          tunnel: w2022 -> [_]
          frame #0 {
            # "set paramaters (rate, volume) for flush, clear volume"
            n1439 = local write "Inject Pump 1"(TRUE ("Inject Pump 1")) -> ()
            n1440 = Number To Decimal String(number="Flush rate (uL/m) P1") -> (decimal integer string=w2048:string)  [unwired: 1 in]
            n1441 = Concatenate Strings("irate  " ("string"), w2048, " u/m" ("string"), "\r") -> (w2050:string)
            n1442 = VISA Write(VISA resource name=w2025, write buffer=w2050) -> (VISA resource name out=w2046:refnum<visa-resource-name>)  [unwired: 1 in, 2 out]
            n1443 = Reciprocal(x="Flush rate (uL/m) P1") -> (1/x=w2029:dbl)
            n1444 = Number To Decimal String(number="Volume (uL) P1") -> (decimal integer string=w2037:string)  [unwired: 1 in]
            n1445 = Multiply(x="Volume (uL) P1", y=w2029) -> (x*y=w2028:dbl)
            n1446 = Concatenate Strings("tvolume  " ("string"), w2037, " u" ("string"), "\r") -> (w2035:string)
            n1447 = Multiply(x=w2028, y=60.0) -> (x*y=→"HP1 Flush Time (s)":dbl)
            n1448 = VISA Write(VISA resource name=w2046, write buffer=w2035) -> (VISA resource name out=w2034:refnum<visa-resource-name>)  [unwired: 1 in, 2 out]
            n1449 = Concatenate Strings("cvolume" ("string"), "\r") -> (w2033:string)
            n1450 = VISA Write(VISA resource name=w2034, write buffer=w2033) -> (VISA resource name out=w2044:refnum<visa-resource-name>)  [unwired: 1 in, 2 out]
            n1451 = Concatenate Strings("irun" ("string"), "\r") -> (w2042:string)
            n1452 = VISA Write(VISA resource name=w2044, write buffer=w2042) -> (VISA resource name out=w2032:refnum<visa-resource-name>)  [unwired: 1 in, 2 out]
          }
          frame #1 {
            "Flushing P1" <- TRUE ("Flushing P3")
          }
        }
      }
      event "Clear Volume": Value Change {
        n1453 = event-data() -> ()  [unwired: 7 out]
        n1454 = Number To Decimal String(number="Normal volume (mL)") -> (decimal integer string=w2057:string)  [unwired: 1 in]
        n1455 = Concatenate Strings("tvolume " ("string"), w2057, " u" ("string"), "\r") -> (w2054:string)
        n1456 = VISA Write(VISA resource name=w2060, write buffer=w2054) -> (VISA resource name out=w2053:refnum<visa-resource-name>)  [unwired: 1 in, 2 out]
        n1457 = local write "Clear Volume"(FALSE ("Clear Volume")) -> ()
        n1458 = Concatenate Strings("cvolume" ("string"), "\r") -> (w2062:string)
        n1459 = VISA Write(VISA resource name=w2053, write buffer=w2062) -> ()  [unwired: 1 in, 3 out]
      }
      event "Clear Volume P3": Value Change {
        n1460 = event-data() -> ()  [unwired: 7 out]
        n1461 = Concatenate Strings("cvolume" ("string"), "\r") -> (w2068:string)
        n1462 = VISA Write(VISA resource name=w2067, write buffer=w2068) -> ()  [unwired: 1 in, 3 out]
        n1463 = local write "Clear Volume P3"(FALSE ("Clear Volume P3")) -> ()
      }
      event "Clear Volume P1": Value Change {
        n1464 = event-data() -> ()  [unwired: 7 out]
        n1465 = Concatenate Strings("cvolume" ("string"), "\r") -> (w2073:string)
        n1466 = local write "Clear Volume P1"(FALSE ("Clear Volume P1")) -> ()
        n1467 = VISA Write(VISA resource name=w2072, write buffer=w2073) -> ()  [unwired: 1 in, 3 out]
      }
      event "Display On P3": Value Change {
        n1468 = event-data() -> ()  [unwired: 7 out]
        n1469 = Select(t="dim 100", s="Display On P3", f="dim 0") -> (s? t:f=w2079:string)
        n1470 = Concatenate Strings(w2079, "\r") -> (w2081:string)
        n1471 = VISA Write(VISA resource name=w2076, write buffer=w2081) -> ()  [unwired: 1 in, 3 out]
      }
      event "Display On P1": Value Change {
        n1472 = event-data() -> ()  [unwired: 7 out]
        n1473 = Select(t="dim 100", s="Display On P1", f="dim 0") -> (s? t:f=w2086:string)
        n1474 = Concatenate Strings(w2086, "\r") -> (w2088:string)
        n1475 = VISA Write(VISA resource name=w2083, write buffer=w2088) -> ()  [unwired: 1 in, 3 out]
      }
      event "Retract Pump 3": Value Change {
        n1476 = event-data() -> ()  [unwired: 7 out]
        n1477 = local write "Retract Pump 3"(FALSE ("Retract Pump 3")) -> ()
        n1478 = case shown="True" "Retract Pump 3" {
          tunnel: w2090 -> [_ w2093]
          frame False {
          }
          frame True {
            n1479 = Number To Decimal String(number="Retract Rate (mL/m)") -> (decimal integer string=w2111:string)  [unwired: 1 in]
            n1480 = Concatenate Strings("wrate  " ("string"), w2111, " u/m" ("string"), "\r") -> (w2113:string)
            n1481 = VISA Write(VISA resource name=w2093, write buffer=w2113) -> (VISA resource name out=w2104:refnum<visa-resource-name>)  [unwired: 1 in, 2 out]
            n1482 = Number To Decimal String(number="Retract Vol 3 (uL)") -> (decimal integer string=w2106:string)  [unwired: 1 in]
            n1483 = Concatenate Strings("tvolume  " ("string"), w2106, " u" ("string"), "\r") -> (w2103:string)
            n1484 = VISA Write(VISA resource name=w2104, write buffer=w2103) -> (VISA resource name out=w2099:refnum<visa-resource-name>)  [unwired: 1 in, 2 out]
            n1485 = Concatenate Strings("cvolume" ("string"), "\r") -> (w2100:string)
            n1486 = VISA Write(VISA resource name=w2099, write buffer=w2100) -> (VISA resource name out=w2094:refnum<visa-resource-name>)  [unwired: 1 in, 2 out]
            n1487 = Concatenate Strings("wrun" ("string"), "\r") -> (w2095:string)
            n1488 = VISA Write(VISA resource name=w2094, write buffer=w2095) -> ()  [unwired: 1 in, 3 out]
          }
        }
      }
      event "Retract Pump 1": Value Change {
        n1489 = event-data() -> ()  [unwired: 7 out]
        n1490 = local write "Retract Pump 1"(FALSE ("Retract Pump 1")) -> ()
        n1491 = case shown="True" "Retract Pump 1" {
          tunnel: w2115 -> [_ w2120]
          frame False {
          }
          frame True {
            n1492 = local read "Retract Rate (mL/m)"() -> (w2118:dbl)
            n1493 = Number To Decimal String(number=w2118) -> (decimal integer string=w2136:string)  [unwired: 1 in]
            n1494 = Concatenate Strings("wrate  " ("string"), w2136, " u/m" ("string"), "\r") -> (w2138:string)
            n1495 = VISA Write(VISA resource name=w2120, write buffer=w2138) -> (VISA resource name out=w2130:refnum<visa-resource-name>)  [unwired: 1 in, 2 out]
            n1496 = Number To Decimal String(number="Retract Vol 1 (uL)") -> (decimal integer string=w2132:string)  [unwired: 1 in]
            n1497 = Concatenate Strings("tvolume  " ("string"), w2132, " u" ("string"), "\r") -> (w2129:string)
            n1498 = VISA Write(VISA resource name=w2130, write buffer=w2129) -> (VISA resource name out=w2126:refnum<visa-resource-name>)  [unwired: 1 in, 2 out]
            n1499 = Concatenate Strings("cvolume" ("string"), "\r") -> (w2127:string)
            n1500 = VISA Write(VISA resource name=w2126, write buffer=w2127) -> (VISA resource name out=w2121:refnum<visa-resource-name>)  [unwired: 1 in, 2 out]
            n1501 = Concatenate Strings("wrun" ("string"), "\r") -> (w2122:string)
            n1502 = VISA Write(VISA resource name=w2121, write buffer=w2122) -> ()  [unwired: 1 in, 3 out]
          }
        }
      }
      event "Flip Green Filter": Value Change {
        n1503 = event-data() -> ()  [unwired: 7 out]
        n1504 = Not(x="Flip Green Filter") -> (.not. x?=w2140:bool)
        n1505 = local write "Flip Green Filter"(w2140) -> ()
        n1506 = flat-sequence {
          tunnel: w2148 -> [w2153]
          tunnel: w2147 -> [w2152]
          tunnel: [w2150] -> w2145
          tunnel: [w2149] -> w2144
          tunnel: [w2155] -> w2143
          tunnel: w2145 -> [w2155]
          tunnel: [w2154] -> w2142
          tunnel: w2144 -> [w2154]
          tunnel: w2143 -> [w2159]
          tunnel: w2142 -> [w2158]
          tunnel: [w2157] -> w2146
          frame #0 {
            n1507 = xnode "Read/Write Control"("FPGA VI Reference In"=w2153, "error in"=w2152, "Green Filter Flipper"=TRUE) -> ("FPGA VI Reference Out"=w2150:T19, "error out"=w2149:errorcluster)
          }
          frame #1 {
            n1508 = Wait (ms)(milliseconds to wait=u32 100) -> ()  [unwired: 1 out]
          }
          frame #2 {
            n1509 = xnode "Read/Write Control"("FPGA VI Reference In"=w2159, "error in"=w2158, "Green Filter Flipper"=FALSE) -> ("error out"=w2157:errorcluster)  [unwired: 1 out]
          }
        }
      }
      event "Pump 1 contents", "Pump 3 contents": Value Change {
        n1510 = event-data() -> ()  [unwired: 7 out]
        n1511 = local read "Pump 1 contents"() -> (→"Pump 1 cont disp":string)
        n1512 = local read "Pump 3 contents"() -> (→"Pump 3 cont disp":string)
      }
      event "Reset Trap Pos. FB": Value Change {
        n1513 = event-data() -> ()  [unwired: 7 out]
        n1514 = xnode "Read/Write Control"("FPGA VI Reference In"=w2165, "error in"=w2164, "Trap Pos. FB Reset"="Reset Trap Pos. FB") -> ()  [unwired: 2 out]
      }
      event "Rem fb disp offset": Value Change {
        n1515 = event-data() -> ()  [unwired: 7 out]
        n1516 = local write "Rem fb disp offset"(FALSE ("Rem fb disp offset")) -> ()
        n1517 = local read "Mean T1 Position (nm)"() -> (w2167:dbl)
        n1518 = local read "FB Trap Pos Offset"() -> (w2168:dbl)
        n1519 = Subtract(x=w2168, y=w2167) -> (x-y=w2166:dbl)
        n1520 = local write "FB Trap Pos Offset"(w2166) -> ()
      }
      event "Threshold (nm)": Value Change {
        n1521 = event-data() -> ()  [unwired: 7 out]
        n1522 = flat-sequence {
          tunnel: w2172 -> [w2180]
          tunnel: w2171 -> [w2179]
          tunnel: [w2173] -> w2170
          tunnel: w2170 -> [w2186]
          frame #0 {
            n1523 = xnode "Read/Write Control"("FPGA VI Reference In"=w2180, "error in"=w2179) -> ("FPGA VI Reference Out"=w2176:T19, "error out"=w2175:errorcluster, "FPGA TTrig Thresh"=w2177:i64)
            n1524 = local read "Threshold stored (nm)"() -> (w2185:dbl)
            n1525 = local read "Threshold (nm)"() -> (w2173:dbl)
            n1526 = local read "AOM X Cal (nm/MHz)"() -> (w2183:dbl)
            n1527 = Subtract(x=w2173, y=w2185) -> (x-y=w2184:dbl)
            n1528 = Divide(x=w2184, y=w2183) -> (x/y=w2181:dbl)
            n1529 = call "IR AOM freq to word.vi"("Frequency In (MHz)"=w2181) -> ("Frequency Word Out (double)"=w2182:dbl)
            n1530 = To Quad Integer(1:w2182) -> (0:w2178:i64)
            n1531 = Add(x=w2177, y=w2178) -> (x+y=w2174:i64)
            n1532 = xnode "Read/Write Control"("FPGA VI Reference In"=w2176, "error in"=w2175, "FPGA TTrig Thresh"=w2174) -> ()  [unwired: 2 out]
          }
          frame #1 {
            "Threshold stored (nm)" <- w2186
          }
        }
      }
      event "FB Trig Integrate": Value Change {
        n1533 = event-data() -> ()  [unwired: 7 out]
        n1534 = local read "FB Trig Integrate"() -> (w2188:u32)
        n1535 = xnode "Read/Write Control"("FPGA VI Reference In"=w2190, "error in"=w2189, "FB Trig Integrate"=w2188) -> ("error out"=w2187:errorcluster)  [unwired: 1 out]
      }
      event "11": Value Change {
        n1536 = event-data() -> ()  [unwired: 7 out]
        n1537 = local read "11"() -> (w2191:bool)
        n1538 = case shown="True" w2191 {
          frame False {
          }
          frame True {
            n1539 = local read "Messages"() -> (w2193:string)
            n1540 = call "Update messages.vi"("Message to add"="You kicked it up to 11!", "Old message string"=w2193) -> ("New message string"=w2194:string)
            n1541 = call <vilib>:"Beep.vi"() -> ()  [unwired: 12 in]
            n1542 = local write "Messages"(w2194) -> ()
          }
        }
      }
      event "Trap Pos. FB ON": Value Change {
        n1543 = event-data() -> ()  [unwired: 7 out]
        n1544 = xnode "Read/Write Control"("FPGA VI Reference In"=w2197, "error in"=w2196, "Force feedback"="Trap Pos. FB ON") -> ()  [unwired: 2 out]
      }
      event "Remove Action Offset": Value Change {
        n1545 = event-data() -> ()  [unwired: 7 out]
        n1546 = local write "Remove Action Offset"(FALSE ("Remove Action Offset")) -> ()
        n1547 = local read "Trap Pos. FB Mult Factor"() -> (w2202:i64)
        n1548 = local read "Trap Pos FB Action"() -> (w2200:i64)
        n1549 = local read "Trap Pos. FB Offset Factor"() -> (w2198:i64)
        n1550 = Multiply(x=w2202, y=w2200) -> (x*y=w2201:i64)
        n1551 = Add(x=w2201, y=w2198) -> (x+y=w2199:i64)
        n1552 = local write "Trap Pos. FB Offset Factor"(w2199) -> ()
        n1553 = xnode "Read/Write Control"("FPGA VI Reference In"=w2205, "error in"=w2204, "Trap Pos. FB Offset Factor"=w2199) -> ()  [unwired: 2 out]
      }
      event "Remove Offset to factor": Value Change {
        n1554 = event-data() -> ()  [unwired: 7 out]
        n1555 = local write "Remove Offset to factor"(FALSE ("Remove Action Offset")) -> ()
        n1556 = local read "Trap Pos. FB Mult Factor"() -> (w2217:i64)
        n1557 = local read "Trap Pos FB Action"() -> (w2215:i64)
        n1558 = local read "Trap Pos. FB Offset Factor"() -> (w2214:i64)
        n1559 = Multiply(x=w2217, y=w2215) -> (x*y=w2216:i64)
        n1560 = local read "Trap Pos. FB Mult Factor"() -> (w2213:i64)
        n1561 = Add(x=w2216, y=w2214) -> (x+y=w2208:i64)
        n1562 = Multiply(x=32768, y="factor") -> (x*y=w2211:dbl)
        n1563 = Multiply(x=w2211, y=w2213) -> (x*y=w2212:dbl)
        n1564 = Subtract(x=w2208, y=w2212) -> (x-y=w2206:dbl)
        n1565 = To Quad Integer(1:w2206) -> (0:w2207:i64)
        n1566 = xnode "Read/Write Control"("FPGA VI Reference In"=w2220, "error in"=w2219, "Trap Pos. FB Offset Factor"=w2207) -> ()  [unwired: 2 out]
